vi "Init Device.vi"(8 "error in (no error)":errorcluster, 11 "Device in":refnum<class "Device.lvclass">) -> (0 "error out":errorcluster, 3 "Device out":refnum<class "Device.lvclass">)   [LabVIEW 2020, in "Device.lvclass"]
uses:
  Device.lvclass
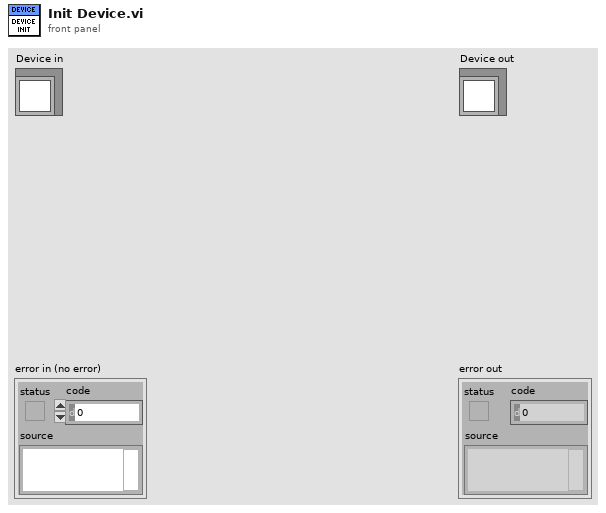
[diagram p1: front panel]
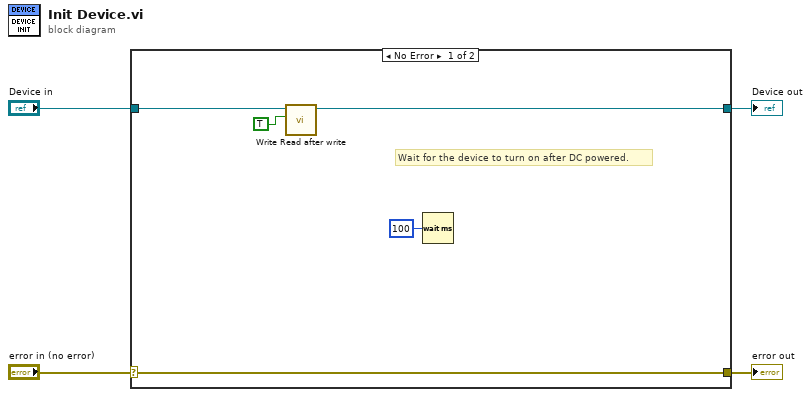
[diagram p0: block diagram]
diagram:
  n1 = case shown="No Error" "error in (no error)" {
    selector: "error in (no error)" -> [w9 w11]
    tunnel: [w9 w11] -> w3
    tunnel: [w6 w10] -> w1
    tunnel: "Device in" -> [w7 w10]
    frame No Error {
      # "Wait for the device to turn on after DC powered."
      n2 = call-dynamic "Write Read after write.vi"("Read after write"=TRUE, "Device in"=w7) -> ("Device out"=w6:refnum<class "Device.lvclass">)  [unwired: 9 in]
      n3 = Wait (ms)(milliseconds to wait=u32 100) -> ()  [unwired: 1 out]
    }
    frame Error {
    }
  }
  "error out" <- w3
  "Device out" <- w1
